vi "TestVI.vi"() -> ()   [LabVIEW 2017]
uses:
  83324dfa-9801-4962-bc77-91914d2e5f01.vi
  cb1c9db4-c671-4eb6-bbe7-2d184d7779db.vi
  8486e2b8-d81d-4fdd-b186-b6ab048937d2.vi
  f78e9434-22aa-4892-a02d-9054408d6bfd.vi
  83324dfa-9801-4962-bc77-91914d2e5f01.vi/6c665dee-f7b0-49ad-9231-125ae7a256b9.vi
  cb1c9db4-c671-4eb6-bbe7-2d184d7779db.vi/6c665dee-f7b0-49ad-9231-125ae7a256b9.vi
  OptionalType/Is Type.vi
  OptionalType/OptionalType.lvclass
panel:
  out "Time with nothing (s)":dbl
  out "O Array":dbl[](array[numeric])
  out "Time with O (s)":dbl
  out "Time with I (s)":dbl
  out "Time with I+O (s)":dbl
  out "I+O Array":dbl[](array[numeric])
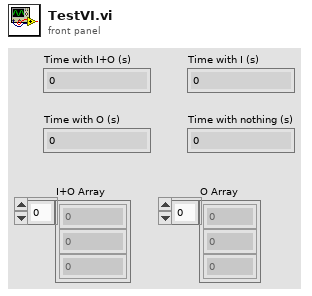
[diagram p1: front panel]
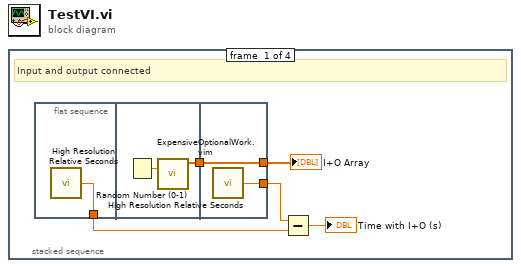
[diagram p0: block diagram]
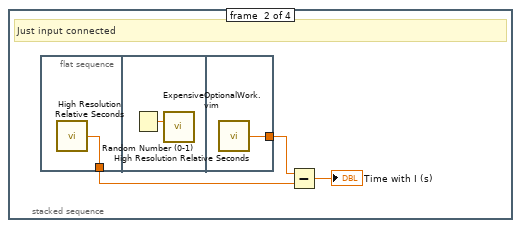
[diagram p2: hidden frame]
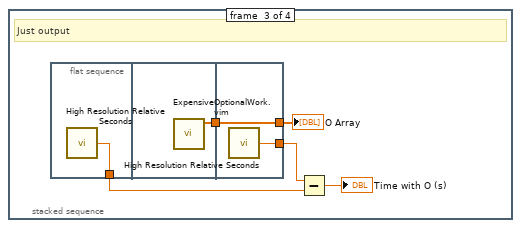
[diagram p3: hidden frame]
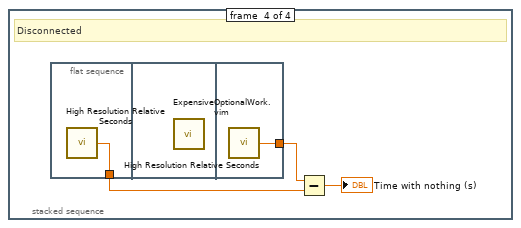
[diagram p4: hidden frame]
diagram:
  n1 = stacked-sequence {
    frame #0 {
      # "Input and output connected"
      n2 = flat-sequence {
        tunnel: [w6] -> w4
        tunnel: [w7] -> w1
        tunnel: [w10] -> w3
        tunnel: [w9] -> w2
        tunnel: w1 -> [w9]
        frame #0 {
          n3 = call <vilib>:"High Resolution Relative Seconds.vi"() -> ("relative seconds"=w6:dbl)
        }
        frame #1 {
          n4 = Random Number (0-1)() -> (number: 0 to 1=w8:dbl)
          n5 = call "ExpensiveOptionalWork.vim"("Optional Input"=w8) -> ("Array"=w7:dbl[])  [unwired: 10 in]
        }
        frame #2 {
          n6 = call <vilib>:"High Resolution Relative Seconds.vi"() -> ("relative seconds"=w10:dbl)
        }
      }
      n7 = Subtract(x=w3, y=w4) -> (x-y=→"Time with I+O (s)":dbl)
      "I+O Array" <- w2
    }
    frame #1 {
      # "Just input connected"
      n8 = flat-sequence {
        tunnel: [w14] -> w12
        tunnel: [w16] -> w11
        frame #0 {
          n9 = call <vilib>:"High Resolution Relative Seconds.vi"() -> ("relative seconds"=w14:dbl)
        }
        frame #1 {
          n10 = Random Number (0-1)() -> (number: 0 to 1=w15:dbl)
          n11 = call "ExpensiveOptionalWork.vim"("Optional Input"=w15) -> ()  [unwired: 10 in, 1 out]
        }
        frame #2 {
          n12 = call <vilib>:"High Resolution Relative Seconds.vi"() -> ("relative seconds"=w16:dbl)
        }
      }
      n13 = Subtract(x=w11, y=w12) -> (x-y=→"Time with I (s)":dbl)
    }
    frame #2 {
      # "Just output"
      n14 = flat-sequence {
        tunnel: [w22] -> w20
        tunnel: [w23] -> w18
        tunnel: [w25] -> w19
        tunnel: [w24] -> w17
        tunnel: w18 -> [w24]
        frame #0 {
          n15 = call <vilib>:"High Resolution Relative Seconds.vi"() -> ("relative seconds"=w22:dbl)
        }
        frame #1 {
          n16 = call "ExpensiveOptionalWork.vim"() -> ("Array"=w23:dbl[])  [unwired: 11 in]
        }
        frame #2 {
          n17 = call <vilib>:"High Resolution Relative Seconds.vi"() -> ("relative seconds"=w25:dbl)
        }
      }
      n18 = Subtract(x=w19, y=w20) -> (x-y=→"Time with O (s)":dbl)
      "O Array" <- w17
    }
    frame #3 {
      # "Disconnected"
      n19 = flat-sequence {
        tunnel: [w29] -> w27
        tunnel: [w30] -> w26
        frame #0 {
          n20 = call <vilib>:"High Resolution Relative Seconds.vi"() -> ("relative seconds"=w29:dbl)
        }
        frame #1 {
          n21 = call "ExpensiveOptionalWork.vim"() -> ()  [unwired: 11 in, 1 out]
        }
        frame #2 {
          n22 = call <vilib>:"High Resolution Relative Seconds.vi"() -> ("relative seconds"=w30:dbl)
        }
      }
      n23 = Subtract(x=w26, y=w27) -> (x-y=→"Time with nothing (s)":dbl)
    }
  }
